vi "phy_dsss_chip_sync.vi"(8 "Threshold":dbl=0.9 format="%#_13g", 11 "dsss_chips":cdb[](array[numeric])) -> (3 "symbols":cdb[](array[numeric]))   [LabVIEW 2014]
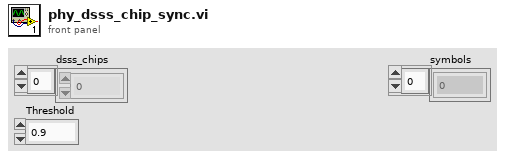
[diagram p1: front panel]
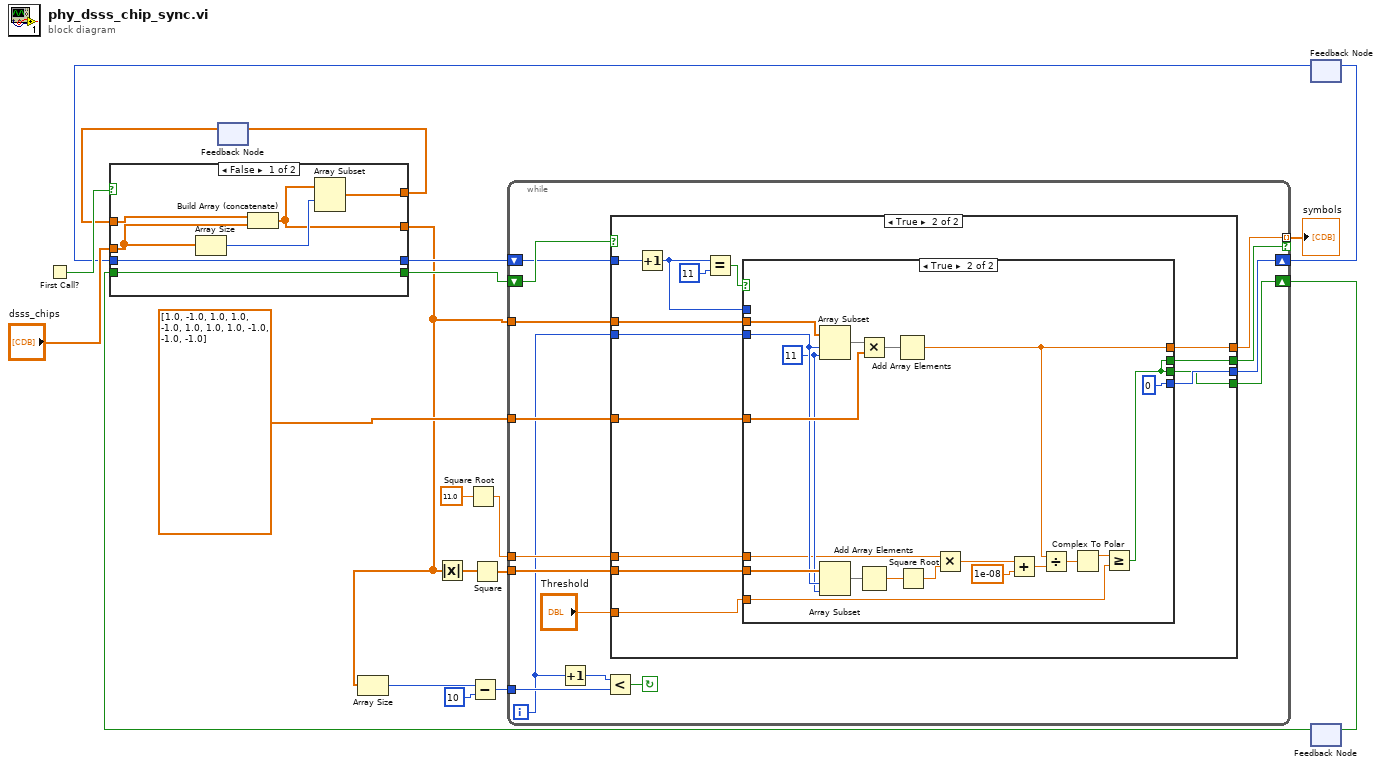
[diagram p0: block diagram]
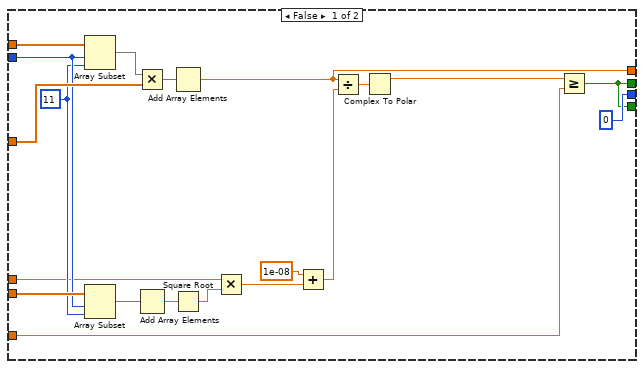
[diagram p2: hidden frame]
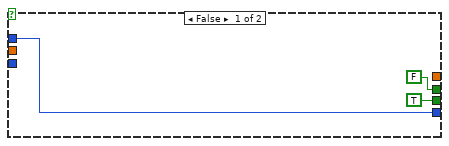
[diagram p3: hidden frame]
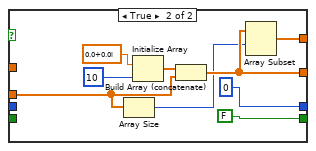
[diagram p4: hidden frame]
diagram:
  n1 = First Call?() -> (First Call?: T/F=w20:bool)
  n2 = feedback #1() -> (w2:cdb[])  [unwired: 1 in]
  n3 = Square Root(x=11.0) -> (sqrt(x)=w4:dbl)
  n4 = feedback #2() -> (w9:i32)  [unwired: 1 in]
  n5 = feedback #3() -> (w11:bool)  [unwired: 1 in]
  n6 = case shown="False" w20 {
    tunnel: "dsss_chips" -> [w24 w30]
    tunnel: [w21 w31] -> w1
    tunnel: [w26 FALSE] -> w18
    tunnel: [w27 0] -> w15
    tunnel: w11 -> [w26 _]
    tunnel: w9 -> [w27 _]
    tunnel: [w22 w28] -> w3
    tunnel: w2 -> [w25 _]
    frame False {
      n7 = Array Size(array=w24) -> (size(s)=w23:i32)
      n8 = Build Array (concatenate)(w25, w24) -> (w21:cdb[])
      n9 = Array Subset(array=w21, index=w23) -> (w22:cdb[])  [unwired: 1 in]
    }
    frame True {
      n10 = Array Size(array=w30) -> (size(s)=w29:i32)
      n11 = Initialize Array(cdb 0.0+0.0i, 10 ("dimension size")) -> (w34:cdb[])
      n12 = Build Array (concatenate)(w34, w30) -> (w31:cdb[])
      n13 = Array Subset(array=w31, index=w29) -> (w28:cdb[])  [unwired: 1 in]
    }
  }
  n14 = feedback-in #1(w3) -> ()
  n15 = Array Size(array=w1) -> (size(s)=w13:i32)
  n16 = Absolute Value(x=w1) -> (abs(x)=w7:dbl[])
  n17 = Subtract(x=w13, y=10) -> (x-y=w16:i32)
  n18 = Square(x=w7) -> (x^2=w6:dbl[])
  n19 = while {
    tunnel: w1 -> [w48]
    shift-right: [w44] -> w12
    shift-left: w18 -> [w49]
    tunnel: w16 -> [w51]
    shift-right: [w45] -> w10
    shift-left: w15 -> [w46]
    tunnel: dbl[] [1.0, -1.0, 1.0, 1.0, -1.0, 1.0, 1.0, 1.0, -1.0, -1.0, -1.0] -> [w47]
    tunnel: [w43] -> w8 mode=indexing if=w42
    tunnel: w6 -> [w40]
    tunnel: w4 -> [w39]
    i -> [w37]
    stop <- w50 continue-if-true
    n20 = Increment(x=w37) -> (x+1=w38:i32)
    n21 = Less?(x=w38, y=w51) -> (x < y?=w50:bool)
    n22 = case shown="True" w49 {
      tunnel: w48 -> [w71 w82]
      tunnel: w37 -> [w62 w81]
      tunnel: w47 -> [w70 w78]
      tunnel: [w53 w77] -> w43
      tunnel: w46 -> [_ w85]
      tunnel: [0 w79] -> w45
      tunnel: [w66 w76] -> w44
      tunnel: [w66 w75] -> w42
      tunnel: "Threshold" -> [w65 w74]
      tunnel: w40 -> [w63 w73]
      tunnel: w39 -> [w57 w72]
      frame False {
        w61 = 11 ("length")
        n23 = Array Subset(array=w71, index=w62, length=w61) -> (w64:cdb[])
        n24 = Array Subset(array=w63, index=w62, length=w61) -> (w60:dbl[])
        n25 = Multiply(x=w64, y=w70) -> (x*y=w68:cdb[])
        n26 = Add Array Elements(numeric array=w60) -> (sum=w59:dbl)
        n27 = Add Array Elements(numeric array=w68) -> (sum=w53:cdb)
        n28 = Square Root(x=w59) -> (sqrt(x)=w58:dbl)
        n29 = Multiply(x=w57, y=w58) -> (x*y=w56:dbl)
        n30 = Add(x=1e-08, y=w56) -> (x+y=w54:dbl)
        n31 = Divide(x=w53, y=w54) -> (x/y=w52:cdb)
        n32 = Complex To Polar(r * e^(i*theta)=w52) -> (r=w69:dbl)  [unwired: 1 out]
        n33 = Greater Or Equal?(x=w69, y=w65) -> (x >= y?=w66:bool)
      }
      frame True {
        n34 = Increment(x=w85) -> (x+1=w80:i32)
        n35 = Equal?(x=w80, y=11) -> (x = y?=w83:bool)
        n36 = case shown="True" w83 {
          tunnel: w82 -> [_ w108]
          tunnel: w81 -> [_ w99]
          tunnel: w80 -> [w88 _]
          tunnel: [w88 0] -> w79
          tunnel: w78 -> [_ w104]
          tunnel: [_ w90] -> w77
          tunnel: [TRUE w103] -> w76
          tunnel: [FALSE w103] -> w75
          tunnel: w74 -> [_ w102]
          tunnel: w73 -> [_ w100]
          tunnel: w72 -> [_ w94]
          frame False {
          }
          frame True {
            w98 = 11 ("length")
            n37 = Array Subset(array=w108, index=w99, length=w98) -> (w101:cdb[])
            n38 = Array Subset(array=w100, index=w99, length=w98) -> (w97:dbl[])
            n39 = Multiply(x=w101, y=w104) -> (x*y=w105:cdb[])
            n40 = Add Array Elements(numeric array=w97) -> (sum=w96:dbl)
            n41 = Add Array Elements(numeric array=w105) -> (sum=w90:cdb)
            n42 = Square Root(x=w96) -> (sqrt(x)=w95:dbl)
            n43 = Multiply(x=w94, y=w95) -> (x*y=w93:dbl)
            n44 = Add(x=w93, y=1e-08) -> (x+y=w91:dbl)
            n45 = Divide(x=w90, y=w91) -> (x/y=w89:cdb)
            n46 = Complex To Polar(r * e^(i*theta)=w89) -> (r=w106:dbl)  [unwired: 1 out]
            n47 = Greater Or Equal?(x=w106, y=w102) -> (x >= y?=w103:bool)
          }
        }
      }
    }
  }
  "symbols" <- w8
  n48 = feedback-in #2(w10) -> ()
  n49 = feedback-in #3(w12) -> ()
